vi "Waveform_Extract from Start and End timestamps.vi"(8 "Error":errorcluster, 9 "Tf Time":timestamp, 10 "T0 Time":timestamp, 11 "Waveform":T1) -> (0 "Error Out":errorcluster, 1 "Tf Out":timestamp, 2 "T0 Out":timestamp, 3 "Waveform Out":T1)   [LabVIEW 2020]
doc: "Retrieves a subset of a waveform at a specified time or index. You must manually select the polymorphic instance you want to use."
uses:
  Universal Controls/Waveform_Data.ctl
  <vilib>/Waveform/WDTOps.llb/WDT Get Final Time Value DBL.vi
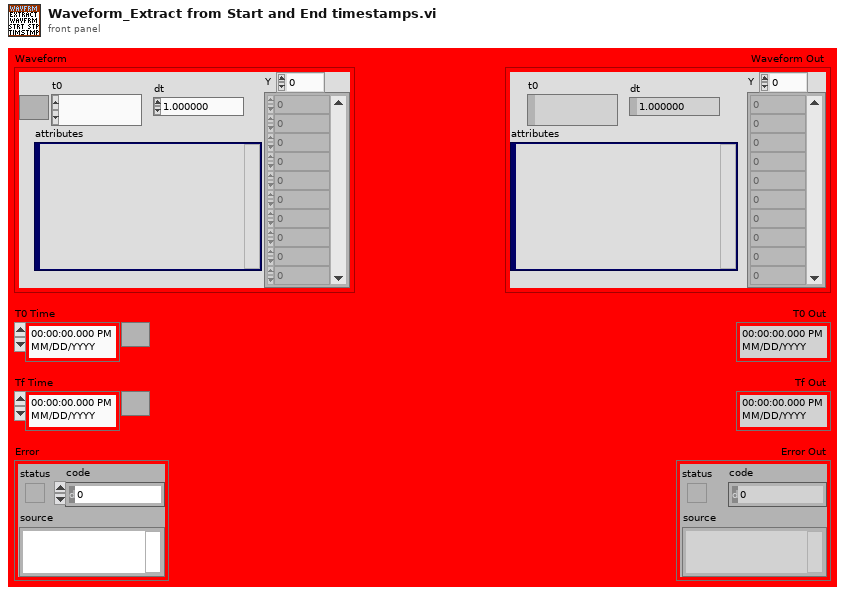
[diagram p1: front panel]
types:
  T1 = typedef "Waveform_Data.ctl" = waveform(dbl)
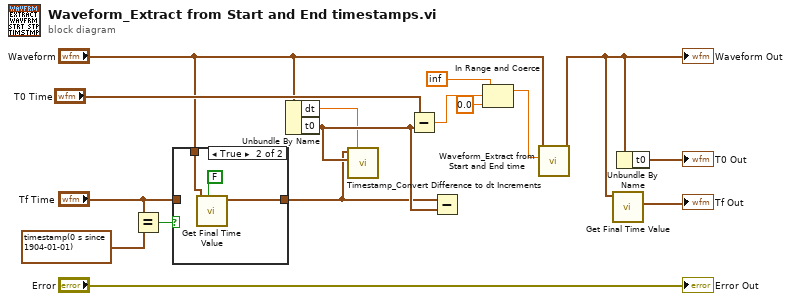
[diagram p0: block diagram]
diagram:
  n1 = Equal?(x="Tf Time", y=timestamp(0 s since 1904-01-01)) -> (x = y?=w7:bool)
  n2 = case shown="True" w7 {
    tunnel: "Waveform" -> [_ w20]
    tunnel: "Tf Time" -> [w17 _]
    tunnel: [w17 w19] -> w2
    frame False {
    }
    frame True {
      n3 = call-poly <vilib>:"Get Final Time Value.vi"("open interval? (T)"=FALSE, "waveform in"=w20) -> ("tf"=w19:timestamp)  [unwired: 7 in, 2 out]
    }
  }
  n4 = Unbundle By Name("Waveform") -> ("dt"=w1:dbl, "t0"=w3:timestamp)
  n5 = call "Timestamp_Convert Difference to dt Increments.vi"("Dt"=w1, "Start Time"=w3, "End Time"=w2) -> ()  [unwired: 6 in, 3 out]
  n6 = Subtract(x="T0 Time", y=w3) -> (x-y=w10:dbl)
  n7 = Subtract(x=w2, y=w3) -> ()  [unwired: 1 out]
  n8 = In Range and Coerce(upper limit=inf, x=w10, lower limit=0.0) -> (coerced(x)=w9:dbl)  [unwired: 1 out]
  n9 = call "Waveform_Extract from Start and End time.vi"("Begin Time"=w9, "Waveform"="Waveform") -> ("Waveform Out"=w15:T1)  [unwired: 6 in, 3 out]
  "Waveform Out" <- w15
  n10 = call-poly <vilib>:"Get Final Time Value.vi"("waveform in"=w15) -> ("tf"=→"Tf Out":timestamp)  [unwired: 8 in, 2 out]
  n11 = Unbundle By Name(w15) -> ("t0"=→"T0 Out":timestamp)
  "Error Out" <- "Error"
